vi "SurreyBALDAS_Local.vi"() -> ()   [LabVIEW 2021]
uses:
  6 Comp Balance Global.vi
panel:
  in  "Quit":bool
  in  "Data Net Button":bool
  in  "data ABS button":bool
  in  "SigConSetup":bool
  in  "Numeric Zero(All Axis) button":bool caption="Numeric Zero(All Axis)"
  out "Roll gauge":dbl(slide) caption="100%             0                -100%" scale=-100.0..100.0
  out "Roll":dbl caption="N.m" format="%#.2f"
  out "Yaw gauge":dbl(slide) caption="100%             0                -100%" scale=-100.0..100.0
  out "Yaw":dbl caption="N.m" format="%#.2f"
  out "Side-force gauge":dbl(slide) caption="100%             0                -100%" scale=-100.0..100.0
  out "Side-Force":dbl caption="N" format="%#.2f"
  out "Drag Gauge":dbl(slide) caption="100%             0                -100%" scale=-100.0..100.0
  out "Drag":dbl caption="N" format="%#.2f"
  out "Pitch gauge":dbl(slide) caption="100%             0                -100%" scale=-100.0..100.0
  out "Pitch":dbl caption="N.m" format="%#.2f"
  out "Lift gauge":dbl(slide) caption="100%             0                -100%" scale=-100.0..100.0
  out "Lift":dbl caption="N" format="%#.2f"
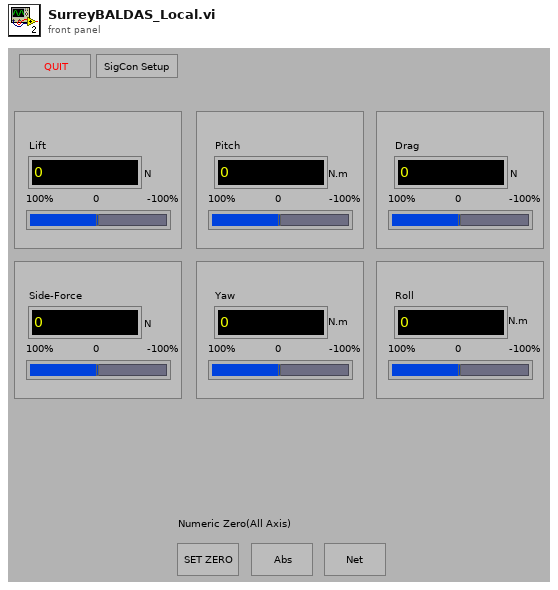
[diagram p1: front panel]
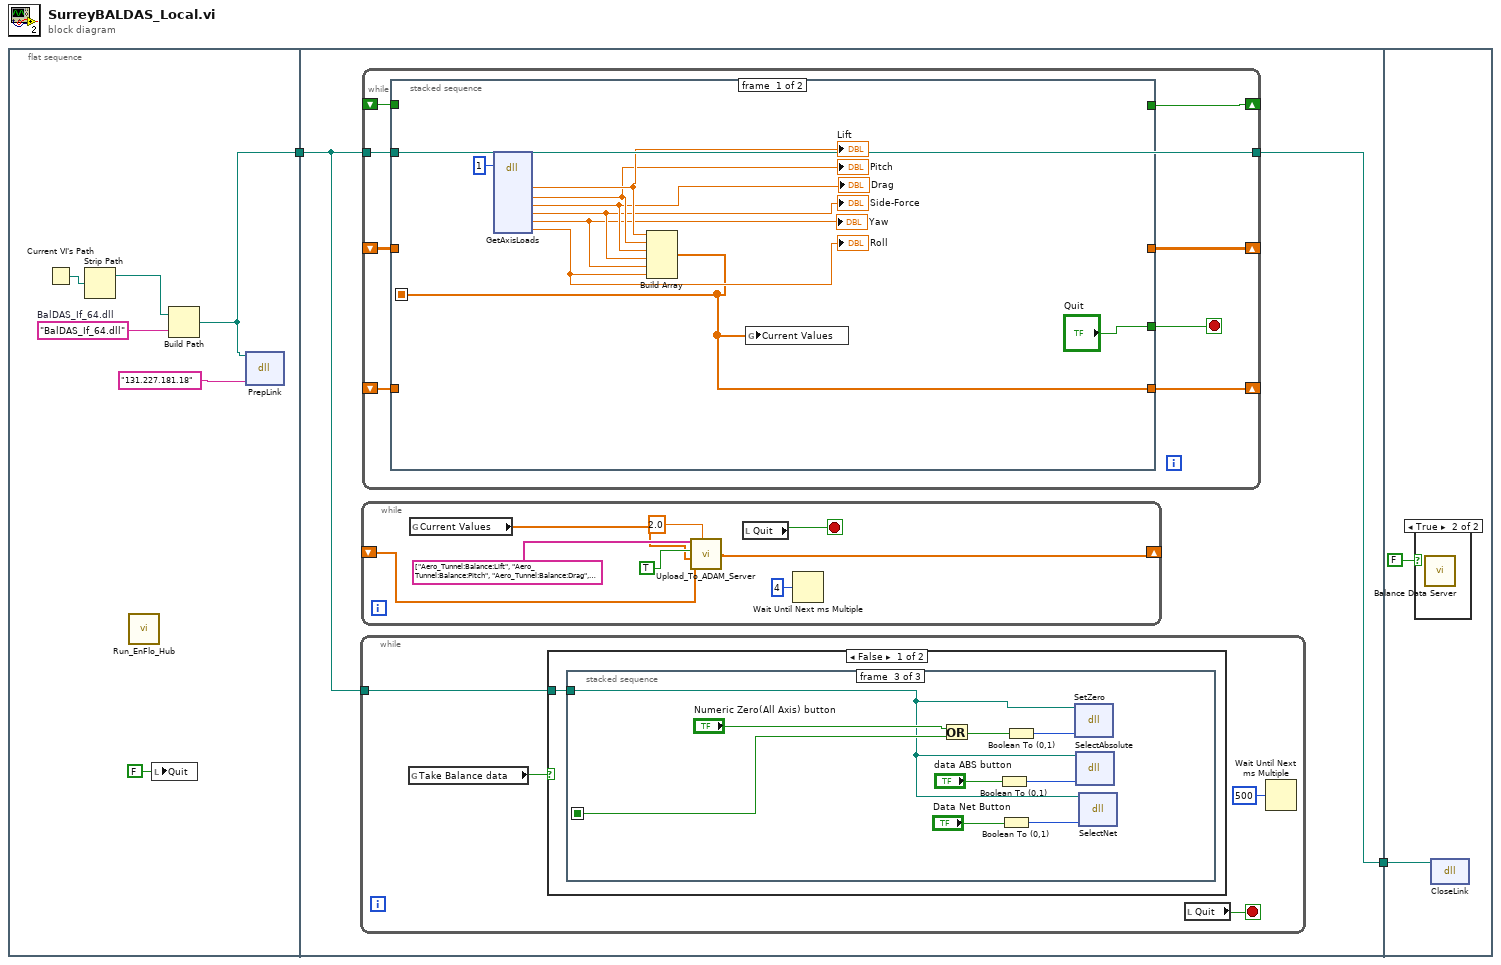
[diagram p0: block diagram]
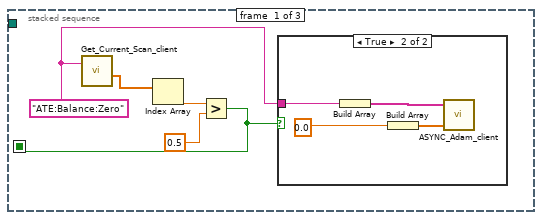
[diagram p2: hidden frame]
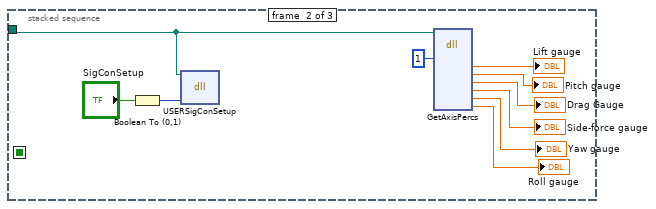
[diagram p4: hidden frame]
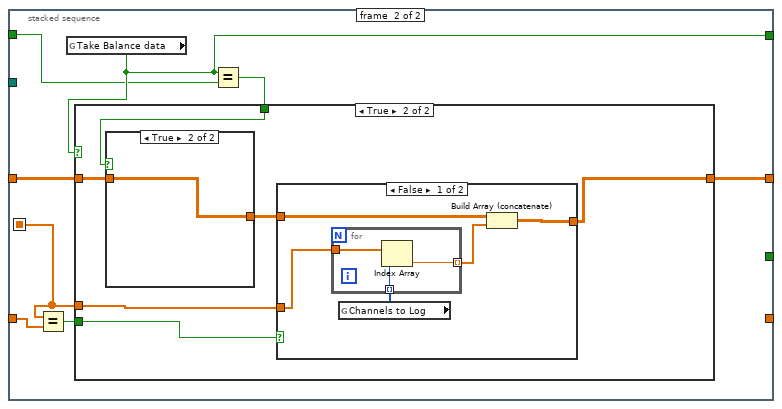
[diagram p6: hidden frame]
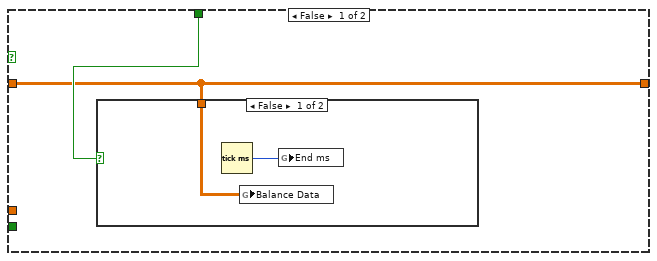
[diagram p7: hidden frame]
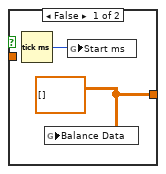
[diagram p9: hidden frame]
diagram:
  n1 = flat-sequence {
    tunnel: [w5] -> w2
    tunnel: w2 -> [w9]
    tunnel: [w10] -> w1
    tunnel: w1 -> [w101]
    frame #0 {
      w4 = "BalDAS_If_64.dll"  # BalDAS_If_64.dll
      n2 = Current VI's Path() -> (path=w7:path)
      n3 = Strip Path(path=w7) -> (stripped path=w6:path)  [unwired: 1 out]
      n4 = call "Run_EnFlo_Hub.vi"() -> ()  [unwired: 7 in, 1 out]
      n5 = local write "Quit"(FALSE ("Quit")) -> ()
      n6 = Build Path(base path=w6, name or relative path=w4) -> (appended path=w5:path)
      n7 = dll-call lib="C:/Aerotech/SurreyBaldas/BalDAS_If.dl" fn="PrepLink"(path in=w5, "IPAddress"="131.227.181.18") -> ()  [unwired: 2 in, 4 out]
    }
    frame #1 {
      n8 = while {
        tunnel: w9 -> [w14]
        stop <- w11 stop-if-true
        n9 = global read "6 Comp Balance Global.vi" "Take Balance data"() -> (w12:bool)
        n10 = case shown="False" w12 {
          tunnel: w14 -> [w15 _]
          frame False {
            n11 = stacked-sequence {
              seq-local: [w16 _ _] -> [_ _ w36]
              tunnel: w15 -> [_ w25 w35]
              frame #0 {
                w18 = "ATE:Balance:Zero"
                n12 = call "Get_Current_Scan_client.vi"("singleChannel"=w18) -> ("Numerical Values"=w19:dbl[])  [unwired: 1 in, 3 out]
                n13 = Index Array(array=w19) -> (element=w20:dbl)  [unwired: 1 in]
                n14 = Greater?(x=w20, y=0.5) -> (0:w16:bool)
                n15 = case shown="True" w16 {
                  tunnel: w18 -> [_ w22]
                  frame False {
                  }
                  frame True {
                    n16 = Build Array(w22) -> (w23:string[])
                    n17 = Build Array(0.0) -> (w24:dbl[])
                    n18 = call "ASYNC_Adam_client.vi"("Values"=w24, "Channel Names"=w23) -> ()  [unwired: 1 in, 2 out]
                  }
                }
              }
              frame #1 {
                n19 = Boolean To (0,1)(Boolean="SigConSetup") -> (0, 1=w33:i16)
                n20 = dll-call lib="C:/Aerotech/SurreyBaldas/BalDAS_If.dl" fn="USERSigConSetup"(path in=w25, "Enable"=w33) -> ()  [unwired: 2 in, 4 out]
                n21 = dll-call lib="C:/Aerotech/SurreyBaldas/BalDAS_If.dl" fn="GetAxisPercs"(path in=w25, "Enable"=1) -> ("Lift"=→"Lift gauge":dbl, "Pitch"=→"Pitch gauge":dbl, "Drag"=→"Drag Gauge":dbl, "side"=→"Side-force gauge":dbl, "Yaw"=→"Yaw gauge":dbl, "Roll"=→"Roll gauge":dbl)  [unwired: 3 in, 9 out]
              }
              frame #2 {
                n22 = Or(x="Numeric Zero(All Axis) button", y=w36) -> (x .or. y?=w43:bool)
                n23 = Boolean To (0,1)(Boolean="data ABS button") -> (0, 1=w41:i16)
                n24 = Boolean To (0,1)(Boolean="Data Net Button") -> (0, 1=w38:i16)
                n25 = Boolean To (0,1)(Boolean=w43) -> (0, 1=w37:i16)
                n26 = dll-call lib="C:/Aerotech/SurreyBaldas/BalDAS_If.dl" fn="SetZero"(path in=w35, "Enable"=w37) -> ()  [unwired: 2 in, 4 out]
                n27 = dll-call lib="C:/Aerotech/SurreyBaldas/BalDAS_If.dl" fn="SelectAbsolute"(path in=w35, "Enable"=w41) -> ()  [unwired: 2 in, 4 out]
                n28 = dll-call lib="C:/Aerotech/SurreyBaldas/BalDAS_If.dl" fn="SelectNet"(path in=w35, "Enable"=w38) -> ()  [unwired: 2 in, 4 out]
              }
            }
          }
          frame True {
          }
        }
        n29 = local read "Quit"() -> (w11:bool)
        n30 = Wait Until Next ms Multiple(millisecond multiple=u32 500) -> ()  [unwired: 1 out]
      }
      n31 = while {
        shift-right: [w48] -> _
        shift-left: _ -> [w47]
        stop <- w45 stop-if-true
        n32 = global read "6 Comp Balance Global.vi" "Current Values"() -> (w46:dbl[])
        n33 = call "Upload_To_ADAM_Server.vi"("Averaging Period (s)"=2.0, "Shift In"=w47, "Channel Values"=w46, "Give Variance"=TRUE, "Channel Names"=string[] ["Aero_Tunnel:Balance:Lift", "Aero_Tunnel:Balance:Pitch", "Aero_Tunnel:Balance:Drag", "Aero_Tunnel:Balance:Side-Force", "Aero_Tunnel:Balance:Yaw", "Aero_Tunnel:Balance:Roll"]) -> ("Shift Out"=w48:dbl[])  [unwired: 1 in]
        n34 = local read "Quit"() -> (w45:bool)
        n35 = Wait Until Next ms Multiple(millisecond multiple=u32 4) -> ()  [unwired: 1 out]
      }
      n36 = while {
        tunnel: w9 -> [w58]
        tunnel: [w58] -> w10
        shift-right: [w56] -> _
        shift-left: _ -> [w57]
        shift-right: [w54] -> _
        shift-left: _ -> [w55]
        shift-right: [w53] -> _
        shift-left: _ -> [w52]
        stop <- w59 stop-if-true
        n37 = stacked-sequence {
          seq-local: [w60 _] -> [_ w71]
          tunnel: ["Quit" _] -> w59
          tunnel: w58 -> [w67 _]
          tunnel: w57 -> [_ w76]
          tunnel: [_ w75] -> w56
          tunnel: w55 -> [_ w73]
          tunnel: [_ w74] -> w54
          tunnel: [w60 _] -> w53
          tunnel: w52 -> [_ w70]
          frame #0 {
            n38 = dll-call lib="C:/Aerotech/SurreyBaldas/BalDAS_If.dl" fn="GetAxisLoads"(path in=w67, "Enable"=1) -> ("Lift"=w66:dbl, "Pitch"=w65:dbl, "Drag"=w64:dbl, "side"=w63:dbl, "Yaw"=w62:dbl, "Roll"=w61:dbl)  [unwired: 3 in, 9 out]
            "Lift" <- w66
            "Pitch" <- w65
            "Drag" <- w64
            "Side-Force" <- w63
            "Yaw" <- w62
            "Roll" <- w61
            n39 = Build Array(w66, w65, w64, w63, w62, w61) -> (w60:dbl[])
            n40 = global write "6 Comp Balance Global.vi" "Current Values"(w60) -> ()
          }
          frame #1 {
            n41 = Equal?(x=w71, y=w70) -> (x = y?=w72:bool)
            n42 = global read "6 Comp Balance Global.vi" "Take Balance data"() -> (w74:bool)
            n43 = Equal?(x=w74, y=w73) -> (x = y?=w77:bool)
            n44 = case shown="True" w74 {
              tunnel: w71 -> [_ w85]
              tunnel: w77 -> [w79 w86]
              tunnel: w76 -> [w78 w84]
              tunnel: [w78 w83] -> w75
              tunnel: w72 -> [_ w82]
              frame False {
                n45 = case shown="False" w79 {
                  tunnel: w78 -> [w80 _]
                  frame False {
                    n46 = Tick Count (ms)() -> (millisecond timer value=w81:u32)
                    n47 = global write "6 Comp Balance Global.vi" "Balance Data"(w80) -> ()
                    n48 = global write "6 Comp Balance Global.vi" "End ms"(w81) -> ()
                  }
                  frame True {
                  }
                }
              }
              frame True {
                n49 = case shown="True" w86 {
                  tunnel: [w88 w90] -> w87
                  tunnel: w84 -> [_ w90]
                  frame False {
                    w88 = dbl[][] [] ("Balance Data")
                    n50 = Tick Count (ms)() -> (millisecond timer value=w89:u32)
                    n51 = global write "6 Comp Balance Global.vi" "Balance Data"(w88) -> ()
                    n52 = global write "6 Comp Balance Global.vi" "Start ms"(w89) -> ()
                  }
                  frame True {
                  }
                }
                n53 = case shown="False" w82 {
                  tunnel: w85 -> [w91 _]
                  tunnel: w87 -> [w95 w99]
                  tunnel: [w92 w99] -> w83
                  frame False {
                    n54 = global read "6 Comp Balance Global.vi" "Channels to Log"() -> (w94:i32[])
                    n55 = for {
                      tunnel: w94 -> [w98] mode=indexing
                      tunnel: w91 -> [w97]
                      tunnel: [w96] -> w93 mode=indexing
                      n56 = Index Array(array=w97, index=w98) -> (element=w96:dbl)
                    }
                    n57 = Build Array (concatenate)(w95, w93) -> (w92:dbl[][])
                  }
                  frame True {
                  }
                }
              }
            }
          }
        }
      }
    }
    frame #2 {
      n58 = case shown="True" FALSE {
        frame False {
        }
        frame True {
          n59 = call "Balance Data Server.vi"() -> ()  [unwired: 9 in, 3 out]
        }
      }
      n60 = dll-call lib="C:/Aerotech/SurreyBaldas/BalDAS_If.dl" fn="CloseLink"(path in=w101) -> ()  [unwired: 2 in, 3 out]
    }
  }
